vi "Cambio_Fecha_Hora.vi"(0 "Cambiar Fecha":bool, 1 "Cambiar hora":bool, 2 "Time":T2 {"Segundo" min=0 max=60; "Minuto" min=0 max=60; "Hora" min=0 max=24}, 3 "Date":T1={"Mes   "=1, "Día         "=1, "Año "=2010} {"Año" min=1900 max=3000 step=1; "Día" min=1 max=31 step=1; "Mes" min=1 max=12 step=1}) -> ()   [LabVIEW 2015]
uses:
  <vilib>/NI_Real-Time Target Support.lvlib
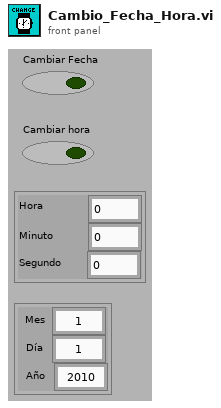
[diagram p1: front panel]
types:
  T1 = cluster{"Mes   ":i32, "Día         ":i32, "Año ":i32}
  T2 = cluster{"Hora        ":i32, "Minuto     ":i32, "Segundo               ":i32}
  T3 = enum16{"set date", "set local time", "set UTC time"}
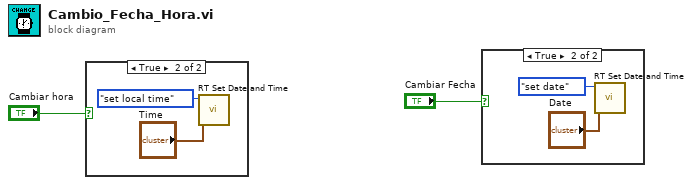
[diagram p0: block diagram]
diagram:
  n1 = case shown="True" "Cambiar hora" {
    frame False {
    }
    frame True {
      n2 = call <vilib>:"RT Set Date and Time.vi"("Time"="Time", "mode"=T3."set local time") -> ()  [unwired: 2 in, 8 out]
    }
  }
  n3 = case shown="True" "Cambiar Fecha" {
    frame False {
    }
    frame True {
      n4 = call <vilib>:"RT Set Date and Time.vi"("Date"="Date", "mode"=T3."set date") -> ()  [unwired: 2 in, 8 out]
    }
  }
